vi "PvgeneratorOP300.vi"(8 "errin":errorcluster, 10 "network":path, 11 "path in":path) -> (0 "sortie d'erreur":errorcluster caption="errout", 1 "network out":path, 2 "tout bon":bool, 3 "Chaîne":string)   [LabVIEW 2020]
uses:
  VG/IS30%.vi
  VG/PN.vi
  <vilib>/Utility/config.llb/NI_LVConfig.lvlib
panel:
  out "nombre de remplacements":i32
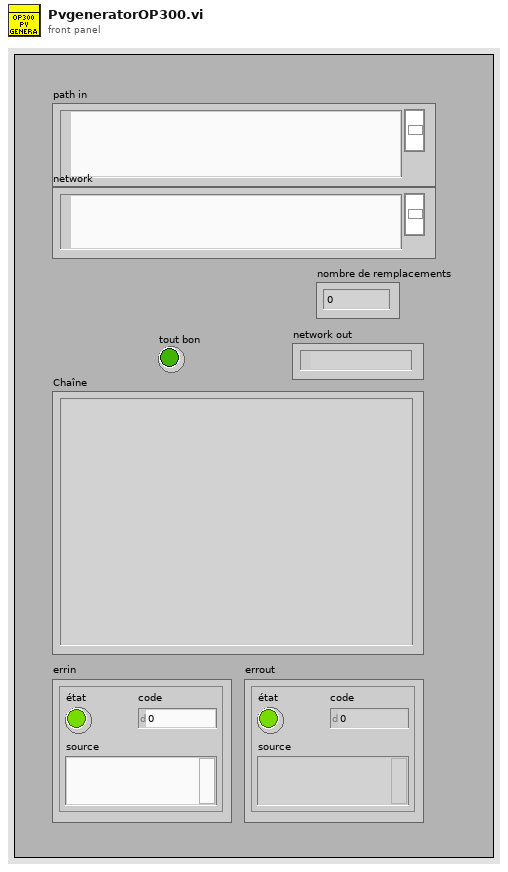
[diagram p1: front panel]
types:
  T1 = enum16{"open", "replace", "create", "open or create", "replace or create", "replace or create with confirmation"}
  T2 = typedef "NI_LVConfig.lvlib/Config Data RefNum.ctl" = refnum<k1>
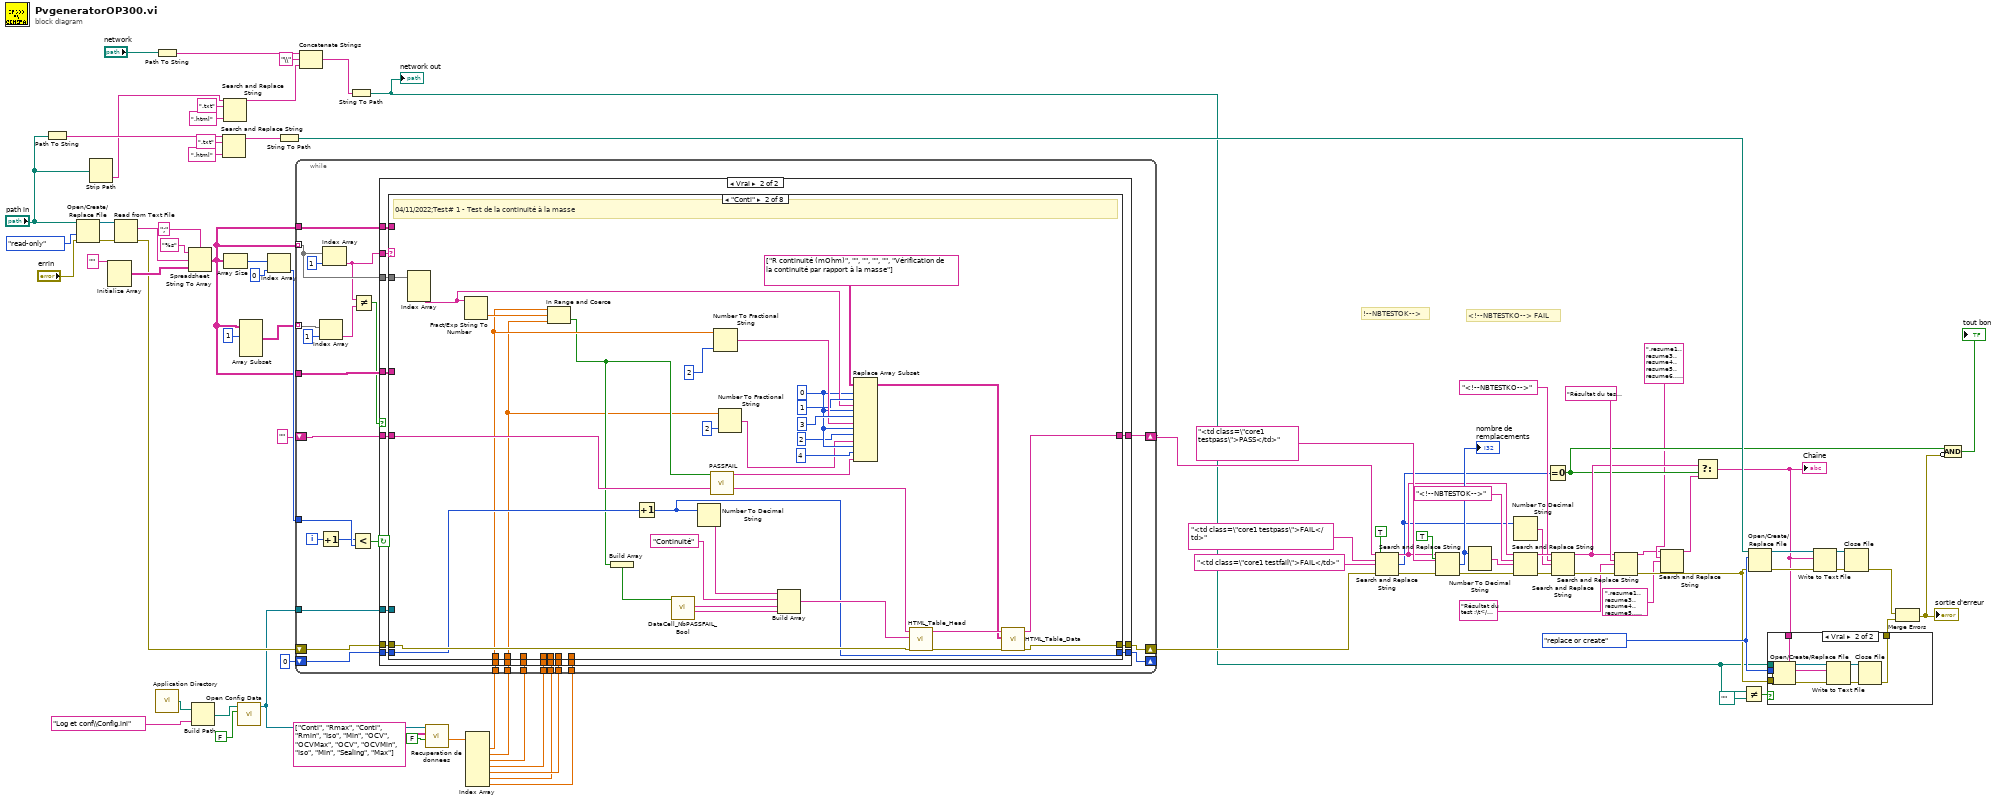
[diagram p0: block diagram]
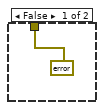
[diagram p2: hidden frame]
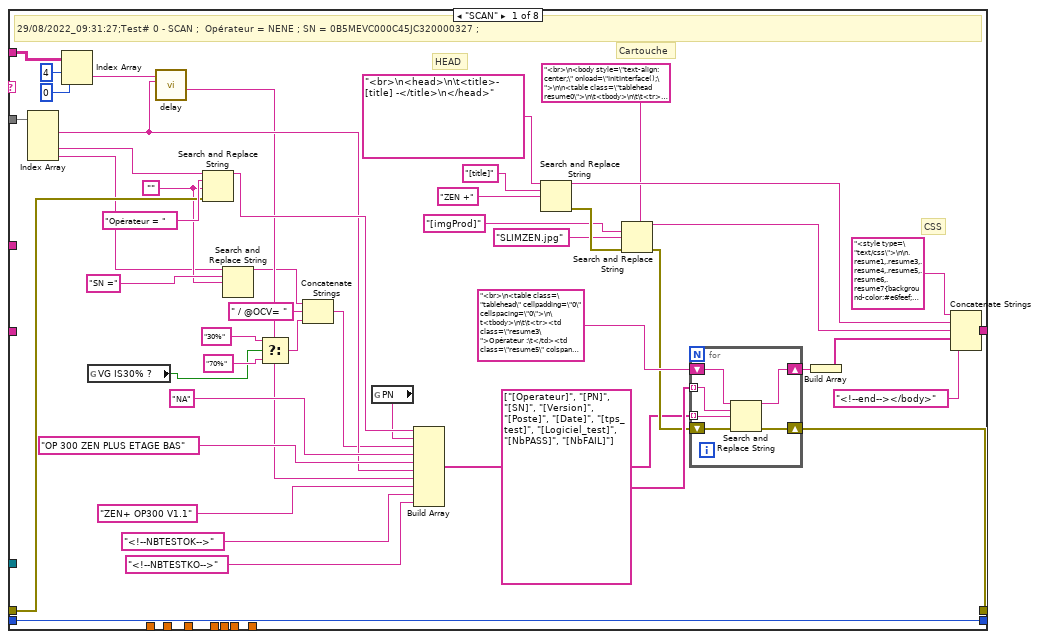
[diagram p4: hidden frame]
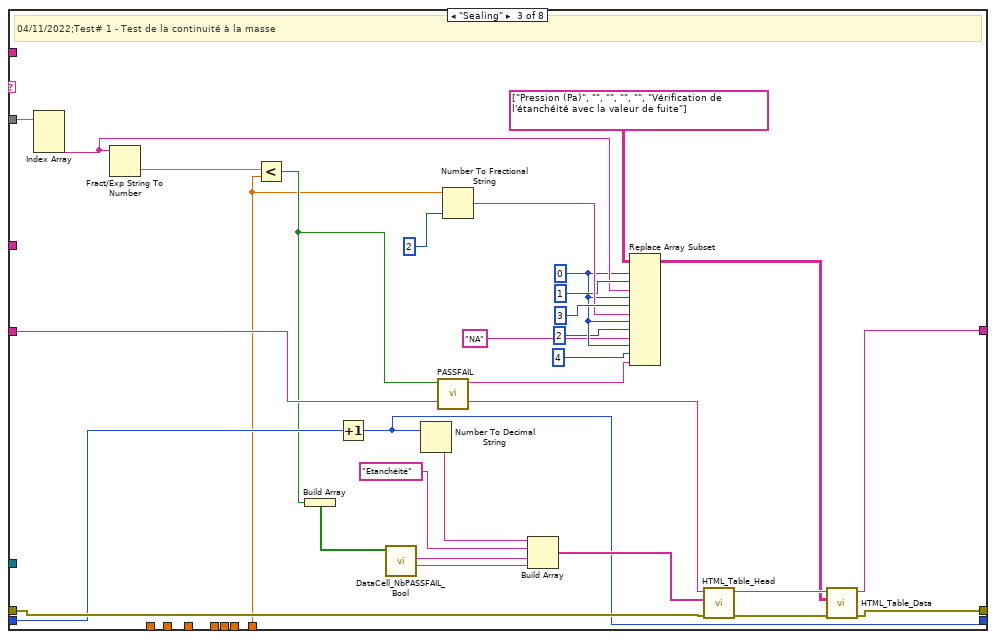
[diagram p5: hidden frame]
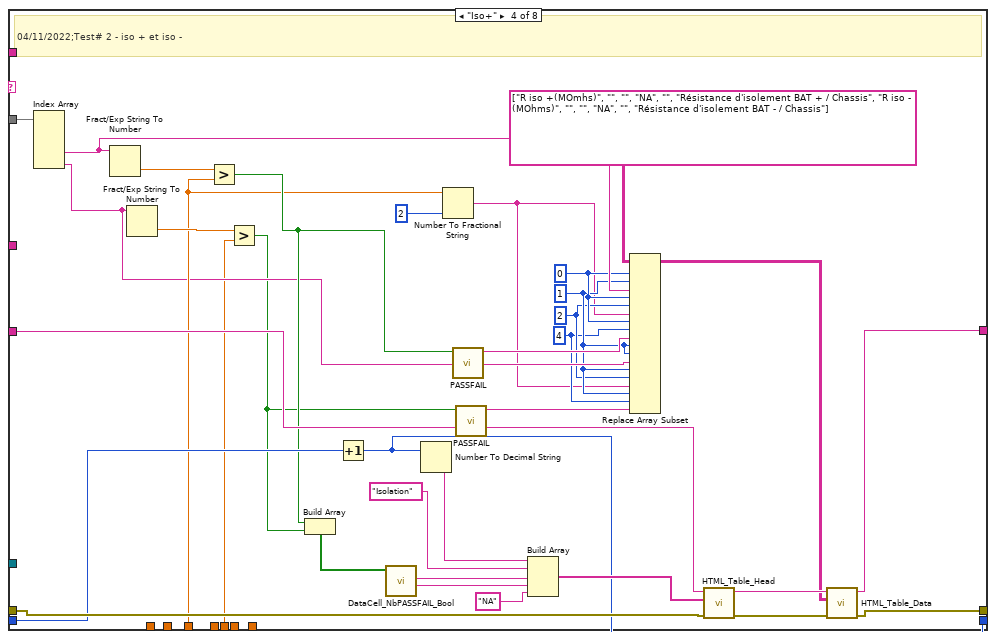
[diagram p6: hidden frame]
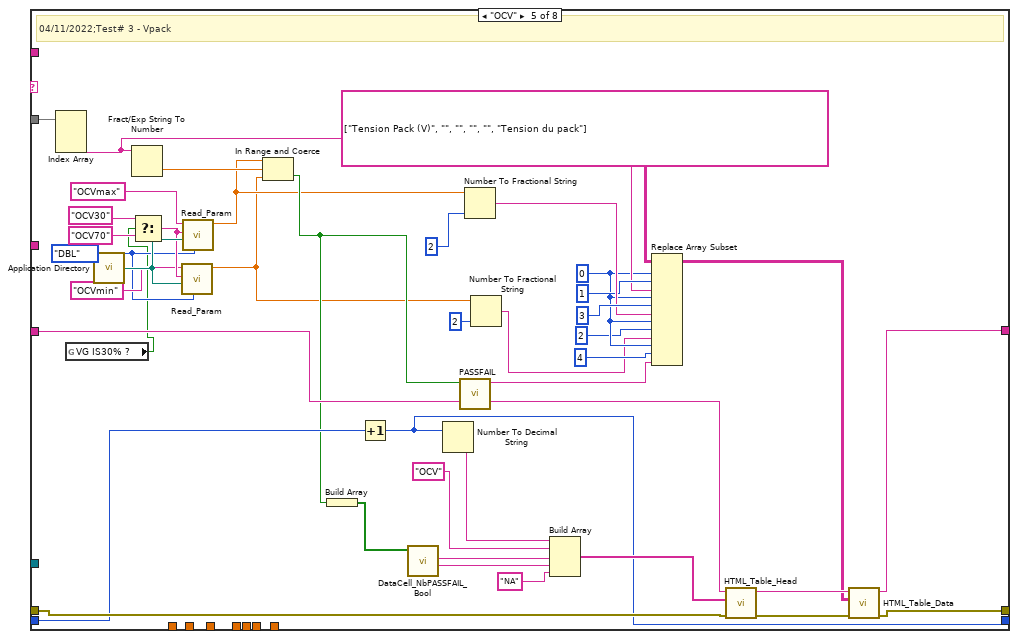
[diagram p7: hidden frame]
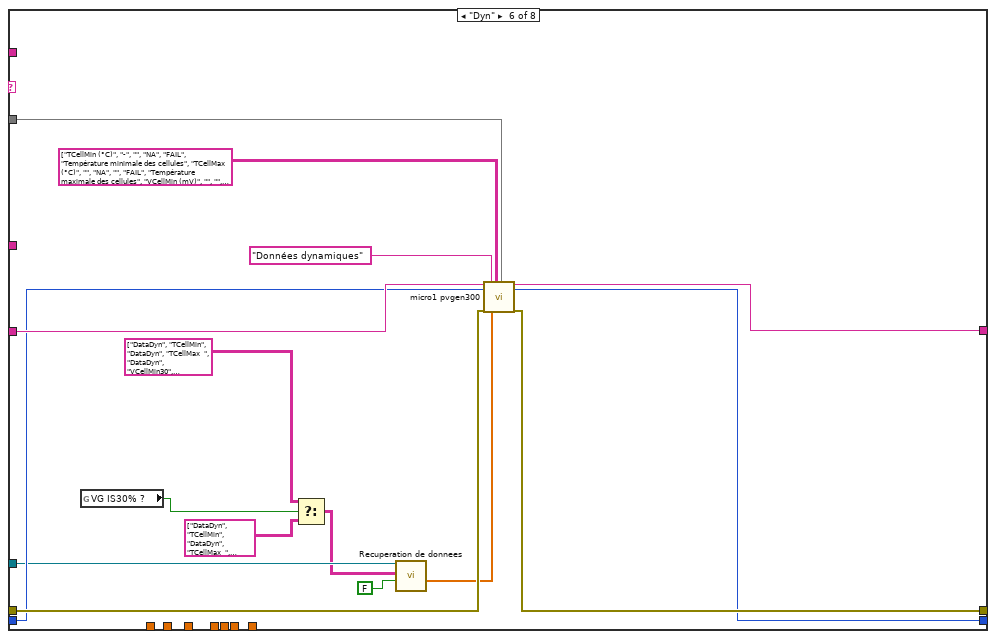
[diagram p8: hidden frame]
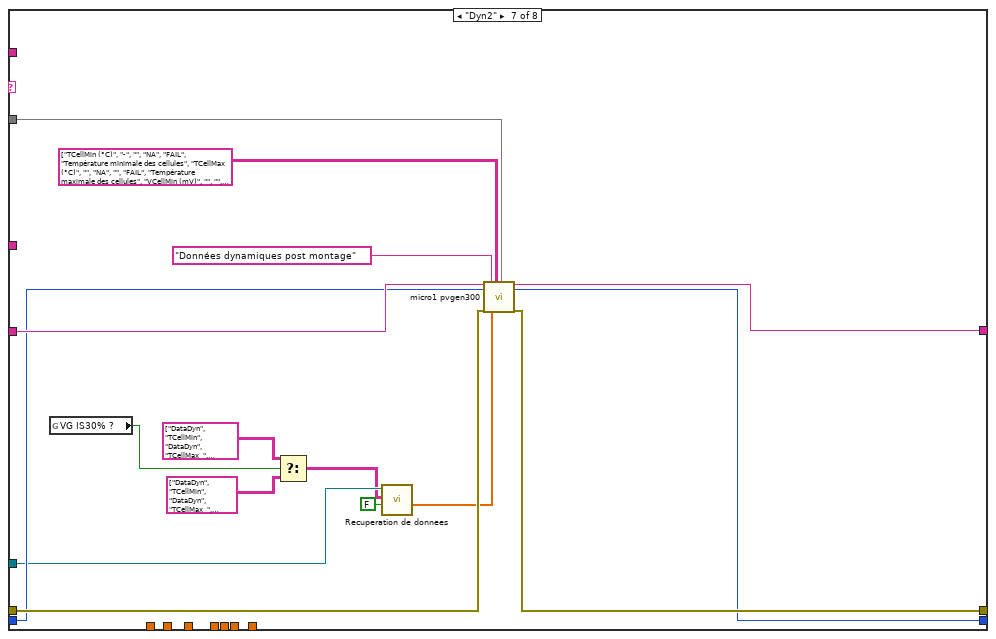
[diagram p9: hidden frame]
diagram:
  w47 = T1."replace or create" ("opération (0 : open)")
  # "<!--NBTESTKO--> FAIL"
  # "!--NBTESTOK-->"
  n1 = Path To String(path="path in") -> (string=w69:string)
  n2 = Open/Create/Replace File(file path (use dialog)="path in", error in="errin", access (0:read/write)=enum16{"read/write", "read-only", "write-only"}."read-only" ("accès (0 : read/write)")) -> (refnum out=w70:refnum<file>, error out=w87:errorcluster)  [unwired: 3 in, 1 out]
  n3 = Strip Path(path="path in") -> (name=w28:string)  [unwired: 1 out]
  n4 = Initialize Array("") -> (w85:string[][])  [unwired: 2 in]
  n5 = Read from Text File(file (use dialog)=w70, error in=w87) -> (text=w83:string, error out=w75:errorcluster)  [unwired: 2 in, 2 out]
  n6 = Path To String(path="network") -> (string=w27:string)
  n7 = call <vilib>:"Application Directory.vi"() -> ("Application Directory"=w19:path)
  n8 = Spreadsheet String To Array(delimiter (Tab)=";" ("séparateur (Tabulation)"), format string="%s" ("chaîne de format"), spreadsheet string=w83, array type (2D Dbl)=w85) -> (array=w6:string[][])
  n9 = Build Path(base path=w19, name or relative path="Log et conf\\Config.ini") -> (appended path=w22:path)
  n10 = Search and Replace String(input string=w69, search string=".txt" ("chaîne recherchée"), replace string=".html" ("chaîne de remplacement (\"\")")) -> (result string=w66:string)  [unwired: 5 in, 3 out]
  n11 = Search and Replace String(input string=w28, search string=".txt" ("chaîne recherchée"), replace string=".html" ("chaîne de remplacement (\"\")")) -> (result string=w25:string)  [unwired: 5 in, 3 out]
  n12 = Array Size(array=w6) -> (size(s)=w81:i32[])
  n13 = call <vilib>:"Open Config Data.vi"("create file if necessary (T)"=FALSE, "configuration file path"=w22) -> ("refnum"=w1:T2)  [unwired: 7 in, 2 out]
  n14 = Array Subset(array=w6, index (row)=1 ("indice")) -> (w4:string[][])  [unwired: 3 in]
  n15 = Index Array(array=w81, index=0 ("indice")) -> (element=w79:i32)
  n16 = String To Path(string=w66) -> (path=w65:path)
  n17 = Concatenate Strings(w27, "\\" ("chaîne"), w25) -> (w24:string)
  n18 = String To Path(string=w24) -> (path=w30:path)
  "network out" <- w30
  n19 = call "Recuperation de donnees.vi"("Est-ce un string?"=FALSE, "Array in"=string[][] [["Conti", "Rmax"], ["Conti", "Rmin"], ["Iso", "Min"], ["OCV", "OCVMax"], ["OCV", "OCVMin"], ["Iso", "Min"], ["Sealing", "Max"]], "Refnum in"=w1) -> ("Array"=w16:dbl[])  [unwired: 7 in, 1 out]
  n20 = Index Array(array=w16) -> (element #1=w15:dbl, element #2=w14:dbl, element #3=w13:dbl, element #4=w12:dbl, element #5=w11:dbl, element #6=w3:dbl, element #7=w2:dbl)  [unwired: 7 in]
  n21 = while {
    tunnel: w79 -> [w114]
    tunnel: w6 -> [w111] mode=indexing
    shift-right: [w110] -> w62
    shift-left: w75 -> [w109]
    shift-right: [w103] -> w64
    shift-left: "" -> [w108]
    shift-right: [w106] -> _
    shift-left: 0 -> [w107]
    tunnel: w6 -> [w105]
    tunnel: w15 -> [w102]
    tunnel: w14 -> [w101]
    tunnel: w6 -> [w100]
    tunnel: w13 -> [w99]
    tunnel: w12 -> [w98]
    tunnel: w11 -> [w97]
    tunnel: w4 -> [w95] mode=indexing
    tunnel: w3 -> [w91]
    tunnel: w2 -> [w90]
    tunnel: w1 -> [w89]
    i -> [w115]
    stop <- w113 continue-if-true
    n22 = Index Array(array=w95, index=1 ("indice")) -> (element=w94:string)
    n23 = Increment(x=w115) -> (x+1=w104:i32)
    n24 = Index Array(array=w111, index=1 ("indice")) -> (element=w93:string)
    n25 = Less?(x=w104, y=w114) -> (x < y?=w113:bool)
    n26 = Not Equal?(x=w93, y=w94) -> (x != y?=w92:bool)
    n27 = case shown="Vrai" w92 {
      tunnel: w111 -> [_ w136]
      tunnel: [w117 w135] -> w110
      tunnel: w109 -> [w117 w134]
      tunnel: w108 -> [w118 w133]
      tunnel: w107 -> [w116 w132]
      tunnel: [w116 w131] -> w106
      tunnel: w105 -> [_ w130]
      tunnel: [w118 w129] -> w103
      tunnel: w93 -> [_ w128]
      tunnel: w102 -> [_ w127]
      tunnel: w101 -> [_ w126]
      tunnel: w100 -> [_ w125]
      tunnel: w99 -> [_ w124]
      tunnel: w98 -> [_ w123]
      tunnel: w97 -> [_ w122]
      tunnel: w91 -> [_ w121]
      tunnel: w90 -> [_ w120]
      tunnel: w89 -> [_ w119]
      frame False {
      }
      frame True {
        n28 = case shown="\"Conti\"" w128 {
          tunnel: w134 -> [w181 w214 w244 w277 w318 w342 w358 w361]
          tunnel: w136 -> [w183 w215 w245 w278 w319 w339 w355 _]
          tunnel: [w160 w213 w243 w276 w317 w341 w357 w361] -> w135
          tunnel: w133 -> [_ w212 w242 w275 w316 w338 w354 w359]
          tunnel: w132 -> [w159 w211 w241 w274 w315 w337 w353 w360]
          tunnel: [w159 w210 w240 w273 w314 w336 w352 w360] -> w131
          tunnel: w130 -> [_ _ _ _ _ _ _ _]
          tunnel: [w158 w209 w239 w272 w313 w340 w356 w359] -> w129
          tunnel: w127 -> [_ w198 _ _ _ _ _ _]
          tunnel: w126 -> [_ w191 _ _ _ _ _ _]
          tunnel: w125 -> [w151 _ _ _ _ _ _ _]
          tunnel: w124 -> [_ _ _ w261 _ _ _ _]
          tunnel: w123 -> [_ _ _ _ _ _ _ _]
          tunnel: w122 -> [_ _ _ _ _ _ _ _]
          tunnel: w121 -> [_ _ _ w252 _ _ _ _]
          tunnel: w120 -> [_ _ w222 _ _ _ _ _]
          tunnel: w119 -> [_ _ _ _ _ w335 w351 _]
          frame "SCAN" {
            w154 = ""
            # "Cartouche"
            # "HEAD"
            # "CSS"
            # "29/08/2022_09:31:27;Test# 0 - SCAN ;  Opérateur = NENE ; SN = 0B5MEVC000C45JC320000327 ;"
            n29 = Index Array(array=w183) -> (element #1=w147:string, element #3=w157:string, element #4=w152:string)  [unwired: 4 in, 1 out]
            n30 = Index Array(array=w151, index (row)=4, index (col)=0 ("disabled index (col)")) -> (element=w148:string)
            n31 = global read "IS30%.vi" "VG IS30% ?"() -> (w138:bool)
            n32 = call "delay.vi"("String"=w147, "String 2"=w148) -> ("Delay calculé"=w146:string)  [unwired: 9 in]
            n33 = Search and Replace String(input string=w157, search string="Opérateur = " ("chaîne recherchée"), replace string=w154, error in=w181) -> (result string=w156:string)  [unwired: 4 in, 3 out]
            n34 = Search and Replace String(input string=w152, search string="SN =" ("chaîne recherchée"), replace string=w154) -> (result string=w144:string)  [unwired: 5 in, 3 out]
            n35 = Select(t="30%" ("y"), s=w138, f="70%" ("y")) -> (s? t:f=w141:string)
            n36 = Concatenate Strings(w144, " / @OCV= " ("chaîne"), w141) -> (w143:string)
            n37 = global read "PN.vi" "PN"() -> (w137:string)
            n38 = Build Array(w156, w137, w143, "NA" ("element"), "OP 300 ZEN PLUS ETAGE BAS" ("chaîne"), w147, w146, "ZEN+ OP300 V1.1" ("chaîne"), "<!--NBTESTOK-->" ("chaîne"), "<!--NBTESTKO-->" ("chaîne")) -> (w161:string[])
            n39 = Search and Replace String(input string="<br>\n<head>\n\t<title>- [title] -</title>\n</head>", search string="[title]" ("chaîne recherchée"), replace string="ZEN +" ("Title")) -> (result string=w177:string, error out=w176:errorcluster)  [unwired: 5 in, 2 out]
            n40 = Search and Replace String(input string="<br>\n<body style=\"text-align: center;\" onload=\"InitInterface();\">\n\n<table class=\"tablehead resume0\">\n\t<tbody>\n\t\t<tr>\n\t\t\t<td> <img src=\"[imgProd]\" style=\"width:194px;height:100px\" class=\"left\"></td>\n\t\t\t<td> <div class=\"center\">PROCES VERBAL DE TEST AUTOMATIQUE</div><div class=\"center\">Zen Plus OP 300</div><br class=\"center\"><div class=\"center\">Forseepower</div></td>\n\t\t\t<td> <img src=\"LOGO FORSEE.png\" style=\"width:194px;height:100px\"  class=\"right\"></td>\n\t\t</tr>\n\t</tbody>\n</table>", search string="[imgProd]", replace string="SLIMZEN.jpg" ("imgProd"), error in=w176) -> (result string=w174:string, error out=w171:errorcluster)  [unwired: 4 in, 2 out]
            n41 = for {
              shift-right: [w188] -> w170
              shift-left: "<br>\n<table class=\"tablehead\" cellpadding=\"0\" cellspacing=\"0\">\n\t<tbody>\n\t\t<tr><td class=\"resume3\">Opérateur :\t</td><td class=\"resume5\" colspan=\"3\">[Operateur]</td></tr>\n\t\t<tr><td class=\"resume3\">PN : </td><td class=\"resume5\" colspan=\"3\">[PN]</td></tr>\n\t\t<tr><td class=\"resume3\">SN : </td><td class=\"resume5\" colspan=\"3\">[SN]</td></tr>\n\t\t<tr><td class=\"resume3\">Version : </td><td class=\"resume5\" colspan=\"3\">[Version]</td></tr>\n\t\t<tr><td class=\"resume3\">Poste : </td><td class=\"resume5\" colspan=\"3\">[Poste]</td></tr>\t\t\n\t\t<tr><td class=\"resume3\">Date du test : </td><td class=\"resume5\" colspan=\"3\">[Date]</td></tr>\n\t\t<tr><td class=\"resume3\">Temps de test : </td><td class=\"resume5\" colspan=\"3\">[tps_test]</td></tr>\n\t\t<tr><td class=\"resume3\">Logiciel de test :\t</td><td class=\"resume5\" colspan=\"3\">[Logiciel_test]</td></tr>\n\t\t<tr><td class=\"resume3\">Résultat du test :\t</td><td class=\"resume5\" colspan=\"3\"><div><span style=\"float:left\" id=\"result\"><font size = \"5pt\" color=\"green\"><b>CONFORME</b></font><b><font size = \"5pt\"> ( </font><font size = \"5pt\" color=\"green\">[NbPASS] PASS </font>  <font size = \"5pt\"> / </font><font size = \"5pt\" color=\"red\">[NbFAIL] FAIL</font> <font size = \"5pt\"> ) </font></b></span></div></td></tr>\n\t</tbody>\n</table>" -> [w189]
              tunnel: string[] ["[Operateur]", "[PN]", "[SN]", "[Version]", "[Poste]", "[Date]", "[tps_test]", "[Logiciel_test]", "[NbPASS]", "[NbFAIL]"] -> [w185] mode=indexing
              tunnel: w161 -> [w184] mode=indexing
              shift-right: [w186] -> w160
              shift-left: w171 -> [w187]
              n42 = Search and Replace String(input string=w189, search string=w185, replace string=w184, error in=w187) -> (result string=w188:string, error out=w186:errorcluster)  [unwired: 4 in, 2 out]
            }
            n43 = Build Array(w170) -> (w169:string[])
            n44 = Concatenate Strings("<style type=\"text/css\">\n\n.resume1,.resume3,.resume4,.resume5,.resume6,.resume7{background-color:#e6feef;padding:7px;border:1px solid black;}\n.resume0{border:1px solid black;background-color:#e6feef;font-weight: bold;padding:0px;text-align: center;}\n.resume1{width:350px;text-align:right;font-weight:bold;}\n.resume3{width:350px;text-align:right;border-top:0px solid black;font-weight:bold;}\n.resume4{border-left:0px solid black;width:290px;}\n.resume5{width:290px;border-left:0px solid black;border-top:0px solid black;}\n.resume6{border-left:0px solid black;width:60px;}\n.resume7{border-left:0px solid black;border-top:0px solid black;width:60px;}\n.title1{text-align: left;background-color:#e6f4fe;padding:10px;border:1px solid #101010;}\n.title2{width: 30px;text-align: center;background-color:#e6f4fe;padding:1px;border:1px solid #101010;border-left:0px solid black;font-weight: bold;}\n.title2 a:link{text-decoration:none;}\n.entete0,.entete1,.entete2,.time2{text-align: center;background-color:#feeec9;padding:7px;border:1px solid black;font-weight: bold;}\n.entete0{width:45px;border-right:0px solid black;}\n.entete1{width:505px;}\n.entete2{width:95px;border-right:0px solid black;}\n.time2{border-left:0px solid black;width:145px;font-size:11px;}\n.core0,.core1,.core2,.core3,.core4,.time{text-align: center;background-color:#fafed3;padding:7px;border:1px solid black;}\n.core0, .core1,.core3,.core4{width:95px;border-top:0px solid black;border-right:0px solid black;}\n.core0{width:45px;}\n.core2{border-top:0px solid black;width:505px;}\n.core3{width:200px;}\n.core4{width:300px;}\n.time{width:145px;border-top:0px solid black;border-left:0px solid black;font-size:11px;}\n.false .core0,.false .core1,.false .core2,.false .core3,.false .core4,.false .time{background-color:#f4f4f4;}\n.false .entete0,.false .entete1,.false .entete2,.false .time2{background-color:#dadada;}\n.false .title1,.false .title2,.false .resultentete .testpass,.false .resultentete .testfail,.false .resultentete .testtime{background-color:#c5cac9;color: blue;}\n.false .title2 a:link{text-decoration:none;color: blue;}\n.comment1,.comment2,.time3{width: 890px;background-color:#e9e8e9;padding:7px;border:1px solid black;border-top:0px solid black;text-align:left;}\n.comment2{border-right:0px solid black;width: 45px;text-align: center;}\n.time3{width: 145px;border-left:0px solid black;font-size:11px;}\n.fixe1{background: -moz-linear-gradient(center top , #101010 10%, #555555 80%) repeat scroll 0 0 transparent;background: -webkit-gradient(linear, left top, left bottom, from(#101010), to(#555555));border:2px solid orange;position : fixed;margin-top:20px;display:none;overflow-y:scroll;max-height:350px;text-shadow: 0px 0px 0 #333333;text-align:left;font-size:10px;padding:10px;margin-left:-162px;border-radius: 15px 15px 15px 15px;}\n.menufixe, .menufixelock{background: -moz-linear-gradient(center top , #101010 80%, transparent 20%) repeat scroll 0 0 transparent;background: -webkit-gradient(linear, left top, left bottom, from(#101010), color-stop(0.65, #101010), to(transparent)) repeat scroll 0 0 transparent;margin: -52px 0px 0px -9px;width:100%;position:fixed;height:55px;-moz-transition: margin 1s;-webkit-transition: margin 1s;}\n.menufixelock, .menufixe:hover{margin: -9px 0px 0px -9px;}\n.lockmenu, .separation,.separationmenu{text-align:center;background: -moz-linear-gradient(center top , #555555 10%, #111111 80%) repeat scroll 0 0 transparent;background: -webkit-gradient(linear, left top, left bottom, from(#555555), to(#111111));border: 1px solid white;border-radius: 10px 10px 10px 10px;box-shadow: 0 -1px 1px #555555 inset;color: #999999;font-weight: bold;width: 100px;padding: 2px;text-decoration: none;}\n.tablehead{width: 1000px;font-family: Verdana;font-size: 12px;margin-left: auto;margin-right: auto;}\n.tablenull{font-family: Verdana;font-size: 11px;margin-left: auto;margin-right: auto;}\n.separationmenu:hover div{display: inline;}\n.lockmenu:hover, .separation:hover,.separationmenu:hover{border: 1px solid orange;cursor:pointer;}\n.lockmenu:hover{border: 1px solid red;cursor:pointer;}\n.separationright{padding:10px;}\ndiv a:link{text-decoration:none;color:#cbcbcb;}\ndiv a:hover{text-decoration:underline;color:#cbcbcb;}\nspan a:link{text-decoration:none;color:#cbcbcb;}\nspan a:hover{text-decoration:none;color:#cbcbcb;}\n.false{color: blue;}\n.testpass{color: green;font-weight: bold;}\n.testfail{color: red;font-weight: bold;}\n.testtime{color: blue;font-weight: bold;}\n.resultentete{font-weight: bold;font-size: 11px;min-width: 200px;text-align:right;}\n.infohard{border: 1px solid black;background-color: white;text-align: center;width: 16px;height: 16px;border-radius: 5px;font-weight: bold;box-shadow: 0 -1px 2px #555555 inset;}\n.infohard:hover{background-color:#feeec9;cursor:pointer;}\n.footerhard{padding-top:30px;}\n.confighard{font-size:10px;width:110px;}\n.circlemain{margin-left:auto;margin-right:auto;}\n.circletext,.circleform{padding-top: 3px;text-align:center;font-size: 10px;width:200px;}\n.circleform{padding-bottom: 3px;padding-top: 1px;}\n.circle{border: 1px solid black;border-collapse: collapse;border-radius: 15px;box-shadow: 1px 1px 0 #505050;height: 15px;width: 15px;display:inline-block;}\n.bookmarkon, .bookmarkoff{background-color: yellow;border: 1px solid black;border-collapse: collapse;border-radius: 10px 10px 10px 10px;box-shadow: 1px 1px 0 #505050;height: 12px;width: 12px;position: absolute;margin-left:22px;cursor: help;}\n.bookmarkoff{background-color: transparent;border: 1px solid #CECECE;box-shadow: none;cursor: copy;}\n.false .bookmarkoff{background-color: transparent;border: 1px solid #E6E1E1;box-shadow: none;cursor: copy;}\n.bookmarkmaster{height: 15px;margin-right: 12px;width: 60px;}\n.bookmarkmaster:hover .bookmarkprev,.bookmarkmaster:hover .bookmarksuiv{display:block;}\n.bookmarkprev, .bookmarksuiv {cursor: pointer;font-size: 25px;font-weight: bold;margin-top: -10px;position: absolute;display:none;}\n.bookmarkprev{margin-left: 2px;}\n.bookmarksuiv{margin-left: 43px;}\n.plus, .moins{background-color: #F4F4F4;border: 1px solid #848484;border-radius: 20px;color: #848484;font-family: arial;font-size: 16px;font-weight: bold;height: 20px;margin-left: 4px;text-align: center;width: 20px;}\n.moins{font-size: 15px;}\n.plus:hover, .moins:hover{background-color: #DADADA;border: 1px solid black;color: black;cursor:pointer;}\n.backtothetop {position: fixed; right: 50%; margin-right: -555px; bottom: 10px; font-size: 35px; font-weight: bold; border: 1px solid #7D7B91; width: 40px; height: 40px; line-height:52px; text-align: center;border-radius: 8px; opacity: 0.25; background-color: #F5F5F5; color:#7D7B91;}\n.backtothetop:hover {opacity: 1; cursor:pointer;}\n.libversion {font-size: 8px;font-weight: normal;padding-right: 10px;text-align: right;}\n.lockmenu {width: 18px;font-size: 12px;}\n.left {display: block; margin-left: 1px;margin-right: auto;}\n.right {display: block; margin-right: 1px;margin-left: auto;}\n.center {display: block; margin-left: auto;margin-right: auto;}\n\n</style>", w177, w174, w169, "<!--end--></body>") -> (w158:string)
          }
          frame "Conti" {
            w195 = 0 ("index (row)")
            # "04/11/2022;Test# 1 - Test de la continuité à la masse"
            n45 = Index Array(array=w215) -> (element #3=w200:string)  [unwired: 3 in, 2 out]
            n46 = Fract/Exp String To Number(string=w200) -> (number=w199:dbl)  [unwired: 3 in, 1 out]
            n47 = In Range and Coerce(upper limit=w198, x=w199, lower limit=w191) -> (In Range?=w193:bool)  [unwired: 1 out]
            n48 = Build Array(w193) -> (w207:bool[])
            n49 = Increment(x=w211) -> (x+1=w210:i32)
            n50 = call <vilib>:"DataCell_NbPASSFAIL_Bool.vi"("Tableau en entrée"=w207) -> ("Chaîne"=w205:string, "Chaîne 2"=w206:string)  [unwired: 8 in, 1 out]
            n51 = Number To Decimal String(number=w210) -> (decimal integer string=w217:string)  [unwired: 1 in]
            n52 = call <vilib>:"PASSFAIL.vi"("E"=w193) -> ("S"=w197:string)  [unwired: 10 in]
            n53 = Number To Fractional String(number=w198, precision (6)=i16 2) -> (F-format string=w203:string)  [unwired: 2 in]
            n54 = Number To Fractional String(number=w191, precision (6)=i16 2) -> (F-format string=w190:string)  [unwired: 2 in]
            n55 = Build Array(w217, "Continuité" ("élément"), w206, w205) -> (w220:string[])
            n56 = Replace Array Subset(array=string[][] [["R continuité (mOhm)", "", "", "", "", "Vérification de la continuité par rapport à la masse"]] ("Tableau"), new element #1=w200, index (row) #1=w195, index (col) #1=1 ("disabled index (col)"), new element #2=w203, index (row) #2=w195, index (col) #2=3 ("disabled index (col)"), new element #3=w190, index (row) #3=w195, index (col) #3=2 ("disabled index (col)"), new element #4=w197, index (row) #4=w195, index (col) #4=4 ("disabled index (col)")) -> (w208:string[][])
            n57 = call "HTML_Table_Head.vi"("entrée d'erreur (pas d'erreur)"=w214, "Tableau"=w220, "chaîne en entrée"=w212) -> ("sortie d'erreur"=w219:errorcluster, "result string"=w218:string)  [unwired: 7 in]
            n58 = call "HTML_Table_Data.vi"("entrée d'erreur (pas d'erreur)"=w219, "Tableau"=w208, "chaîne en entrée"=w218) -> ("sortie d'erreur"=w213:errorcluster, "result string"=w209:string)  [unwired: 7 in]
          }
          frame "Sealing" {
            w226 = 0 ("index (row)")
            # "04/11/2022;Test# 1 - Test de la continuité à la masse"
            n59 = Index Array(array=w245) -> (element #3=w230:string)  [unwired: 3 in, 2 out]
            n60 = Fract/Exp String To Number(string=w230) -> (number=w229:dbl)  [unwired: 3 in, 1 out]
            n61 = Less?(x=w229, y=w222) -> (x < y?=w224:bool)
            n62 = Build Array(w224) -> (w237:bool[])
            n63 = Increment(x=w241) -> (x+1=w240:i32)
            n64 = call <vilib>:"DataCell_NbPASSFAIL_Bool.vi"("Tableau en entrée"=w237) -> ("Chaîne"=w235:string, "Chaîne 2"=w236:string)  [unwired: 8 in, 1 out]
            n65 = Number To Decimal String(number=w240) -> (decimal integer string=w247:string)  [unwired: 1 in]
            n66 = call <vilib>:"PASSFAIL.vi"("E"=w224) -> ("S"=w228:string)  [unwired: 10 in]
            n67 = Number To Fractional String(number=w222, precision (6)=i16 2) -> (F-format string=w233:string)  [unwired: 2 in]
            n68 = Build Array(w247, "Etanchéité" ("élément"), w236, w235) -> (w250:string[])
            n69 = Replace Array Subset(array=string[][] [["Pression (Pa)", "", "", "", "", "Vérification de l'étanchéité avec la valeur de fuite"]] ("Tableau"), new element #1=w230, index (row) #1=w226, index (col) #1=1 ("disabled index (col)"), new element #2=w233, index (row) #2=w226, index (col) #2=3 ("disabled index (col)"), new element #3="NA" ("nouvel élément/sous-tableau"), index (row) #3=w226, index (col) #3=2 ("disabled index (col)"), new element #4=w228, index (row) #4=w226, index (col) #4=4 ("disabled index (col)")) -> (w238:string[][])
            n70 = call "HTML_Table_Head.vi"("entrée d'erreur (pas d'erreur)"=w244, "Tableau"=w250, "chaîne en entrée"=w242) -> ("sortie d'erreur"=w249:errorcluster, "result string"=w248:string)  [unwired: 7 in]
            n71 = call "HTML_Table_Data.vi"("entrée d'erreur (pas d'erreur)"=w249, "Tableau"=w238, "chaîne en entrée"=w248) -> ("sortie d'erreur"=w243:errorcluster, "result string"=w239:string)  [unwired: 7 in]
          }
          frame "Iso+" {
            w256 = 4 ("disabled index (col)")
            w257 = 2 ("disabled index (col)")
            w258 = 1 ("disabled index (col)")
            w265 = 0 ("index (row)")
            # "04/11/2022;Test# 2 - iso + et iso -"
            n72 = Index Array(array=w278) -> (element #3=w266:string, element #5=w259:string)  [unwired: 5 in, 3 out]
            n73 = Fract/Exp String To Number(string=w266) -> (number=w264:dbl)  [unwired: 3 in, 1 out]
            n74 = Fract/Exp String To Number(string=w259) -> (number=w262:dbl)  [unwired: 3 in, 1 out]
            n75 = Greater?(x=w264, y=w261) -> (0:w263:bool)
            n76 = Greater?(x=w262, y=w252) -> (0:w254:bool)
            n77 = Build Array(w263, w254) -> (w270:bool[])
            n78 = Increment(x=w274) -> (x+1=w273:i32)
            n79 = call <vilib>:"DataCell_NbPASSFAIL_Bool.vi"("Tableau en entrée"=w270) -> ("Chaîne"=w268:string, "Chaîne 2"=w269:string)  [unwired: 8 in, 1 out]
            n80 = Number To Decimal String(number=w273) -> (decimal integer string=w281:string)  [unwired: 1 in]
            n81 = Number To Fractional String(number=w261, precision (6)=i16 2) -> (F-format string=w255:string)  [unwired: 2 in]
            n82 = call <vilib>:"PASSFAIL.vi"("E"=w263) -> ("S"=w260:string)  [unwired: 10 in]
            n83 = call <vilib>:"PASSFAIL.vi"("E"=w254) -> ("S"=w253:string)  [unwired: 10 in]
            n84 = Build Array(w281, "Isolation" ("élément"), w269, w268, "NA" ("élément")) -> (w284:string[])
            n85 = Replace Array Subset(array=string[][] [["R iso +(MOmhs)", "", "", "NA", "", "Résistance d'isolement BAT + / Chassis"], ["R iso - (MOhms)", "", "", "NA", "", "Résistance d'isolement BAT - / Chassis"]] ("Tableau"), new element #1=w266, index (row) #1=w265, index (col) #1=w258, new element #2=w255, index (row) #2=w265, index (col) #2=w257, new element #3=w260, index (row) #3=w265, index (col) #3=w256, new element #4=w259, index (row) #4=w258, index (col) #4=w258, new element #5=w255, index (row) #5=w258, index (col) #5=w257, new element #6=w253, index (row) #6=w258, index (col) #6=w256) -> (w271:string[][])
            n86 = call "HTML_Table_Head.vi"("entrée d'erreur (pas d'erreur)"=w277, "Tableau"=w284, "chaîne en entrée"=w275) -> ("sortie d'erreur"=w283:errorcluster, "result string"=w282:string)  [unwired: 7 in]
            n87 = call "HTML_Table_Data.vi"("entrée d'erreur (pas d'erreur)"=w283, "Tableau"=w271, "chaîne en entrée"=w282) -> ("sortie d'erreur"=w276:errorcluster, "result string"=w272:string)  [unwired: 7 in]
          }
          frame "OCV" {
            w289 = enum16{"STR", "DBL", "U32"}."DBL" ("Énum")
            w300 = 0 ("index (row)")
            # "04/11/2022;Test# 3 - Vpack"
            n88 = Index Array(array=w319) -> (element #3=w304:string)  [unwired: 3 in, 2 out]
            n89 = global read "IS30%.vi" "VG IS30% ?"() -> (w286:bool)
            n90 = call <vilib>:"Application Directory.vi"() -> ("Application Directory"=w293:path)
            n91 = Fract/Exp String To Number(string=w304) -> (number=w303:dbl)  [unwired: 3 in, 1 out]
            n92 = Select(t="OCV30" ("section"), s=w286, f="OCV70" ("section")) -> (s? t:f=w292:string)
            n93 = call "Read_Param.vi"("Énum"=w289, "pathin"=w293, "section"=w292, "key"="OCVmin") -> ("dbl"=w287:dbl)  [unwired: 3 in, 4 out]
            n94 = call "Read_Param.vi"("Énum"=w289, "pathin"=w293, "section"=w292, "key"="OCVmax") -> ("dbl"=w288:dbl)  [unwired: 3 in, 4 out]
            n95 = In Range and Coerce(upper limit=w288, x=w303, lower limit=w287) -> (In Range?=w298:bool)  [unwired: 1 out]
            n96 = Build Array(w298) -> (w311:bool[])
            n97 = Increment(x=w315) -> (x+1=w314:i32)
            n98 = call <vilib>:"DataCell_NbPASSFAIL_Bool.vi"("Tableau en entrée"=w311) -> ("Chaîne"=w309:string, "Chaîne 2"=w310:string)  [unwired: 8 in, 1 out]
            n99 = Number To Decimal String(number=w314) -> (decimal integer string=w322:string)  [unwired: 1 in]
            n100 = call <vilib>:"PASSFAIL.vi"("E"=w298) -> ("S"=w302:string)  [unwired: 10 in]
            n101 = Number To Fractional String(number=w288, precision (6)=i16 2) -> (F-format string=w307:string)  [unwired: 2 in]
            n102 = Number To Fractional String(number=w287, precision (6)=i16 2) -> (F-format string=w296:string)  [unwired: 2 in]
            n103 = Build Array(w322, "OCV" ("élément"), w310, w309, "NA" ("élément")) -> (w325:string[])
            n104 = Replace Array Subset(array=string[][] [["Tension Pack (V)", "", "", "", "", "Tension du pack"]] ("Tableau"), new element #1=w304, index (row) #1=w300, index (col) #1=1 ("disabled index (col)"), new element #2=w307, index (row) #2=w300, index (col) #2=3 ("disabled index (col)"), new element #3=w296, index (row) #3=w300, index (col) #3=2 ("disabled index (col)"), new element #4=w302, index (row) #4=w300, index (col) #4=4 ("disabled index (col)")) -> (w312:string[][])
            n105 = call "HTML_Table_Head.vi"("entrée d'erreur (pas d'erreur)"=w318, "Tableau"=w325, "chaîne en entrée"=w316) -> ("sortie d'erreur"=w324:errorcluster, "result string"=w323:string)  [unwired: 7 in]
            n106 = call "HTML_Table_Data.vi"("entrée d'erreur (pas d'erreur)"=w324, "Tableau"=w312, "chaîne en entrée"=w323) -> ("sortie d'erreur"=w317:errorcluster, "result string"=w313:string)  [unwired: 7 in]
          }
          frame "Dyn" {
            n107 = global read "IS30%.vi" "VG IS30% ?"() -> (w328:bool)
            n108 = Select(t=string[][] [["DataDyn", "TCellMin"], ["DataDyn", "TCellMax  "], ["DataDyn", "VCellMin30"], ["DataDyn", "VCellMax30"], ["DataDyn", "TusineMax"], ["DataDyn", "TusineMin"], ["DataDyn", "DeltaT "], ["DataDyn", "DeltaV "]], s=w328, f=string[][] [["DataDyn", "TCellMin"], ["DataDyn", "TCellMax  "], ["DataDyn", "VCellMin70 "], ["DataDyn", "VCellMax70"], ["DataDyn", "TusineMax"], ["DataDyn", "TusineMin"], ["DataDyn", "DeltaT "], ["DataDyn", "DeltaV "]]) -> (s? t:f=w329:string[][])
            n109 = call "Recuperation de donnees.vi"("Est-ce un string?"=FALSE, "Array in"=w329, "Refnum in"=w335) -> ("Array"=w331:dbl[])  [unwired: 7 in, 1 out]
            n110 = call "micro1 pvgen300.vi"("FluxStrIn"=w338, "Numin"=w337, "errin"=w342, "testlabel"="Données dynamiques", "Data limit"=w331, "tab ref"=string[][] [["TCellMin (°C)", "-", "", "NA", "FAIL", "Température minimale des cellules"], ["TCellMax (°C)", "", "NA", "", "FAIL", "Température maximale des cellules"], ["VCellMin (mV)", "", "", "NA", "FAIL", "Tension minimale des cellues"], ["VCellMax (mV)", "", "NA", "", "FAIL", "Tension maximale des cellues"], ["Tusine (°C)", "", "", "", "FAIL", "Température de l'usine"], ["DeltaT (°C)", "", "NA", "", "FAIL", "Différence maximale de température entre les cellules"], ["DeltaV  (mV)", "", "NA", "", "FAIL", "Différence maximale de tension entre les cellules"]] ("Tableau"), "ligne à traiter"=w339) -> ("result string"=w340:string, "Numout"=w336:i32, "errout"=w341:errorcluster)  [unwired: 10 in]
          }
          frame "Dyn2" {
            n111 = global read "IS30%.vi" "VG IS30% ?"() -> (w343:bool)
            n112 = Select(t=string[][] [["DataDyn", "TCellMin"], ["DataDyn", "TCellMax  "], ["DataDyn", "VCellMin30"], ["DataDyn", "VCellMax30"], ["DataDyn", "TusineMax"], ["DataDyn", "TusineMin"], ["DataDyn", "DeltaT "], ["DataDyn", "DeltaV "]], s=w343, f=string[][] [["DataDyn", "TCellMin"], ["DataDyn", "TCellMax  "], ["DataDyn", "VCellMin70 "], ["DataDyn", "VCellMax70"], ["DataDyn", "TusineMax"], ["DataDyn", "TusineMin"], ["DataDyn", "DeltaT "], ["DataDyn", "DeltaV "]]) -> (s? t:f=w345:string[][])
            n113 = call "Recuperation de donnees.vi"("Est-ce un string?"=FALSE, "Array in"=w345, "Refnum in"=w351) -> ("Array"=w344:dbl[])  [unwired: 7 in, 1 out]
            n114 = call "micro1 pvgen300.vi"("FluxStrIn"=w354, "Numin"=w353, "errin"=w358, "testlabel"="Données dynamiques post montage", "Data limit"=w344, "tab ref"=string[][] [["TCellMin (°C)", "-", "", "NA", "FAIL", "Température minimale des cellules"], ["TCellMax (°C)", "", "NA", "", "FAIL", "Température maximale des cellules"], ["VCellMin (mV)", "", "", "NA", "FAIL", "Tension minimale des cellues"], ["VCellMax (mV)", "", "NA", "", "FAIL", "Tension maximale des cellues"], ["Tusine (°C)", "", "", "", "FAIL", "Température de l'usine"], ["DeltaT (°C)", "", "NA", "", "FAIL", "Différence maximale de température entre les cellules"], ["DeltaV  (mV)", "", "NA", "", "FAIL", "Différence maximale de tension entre les cellules"]] ("Tableau"), "ligne à traiter"=w355) -> ("result string"=w356:string, "Numout"=w352:i32, "errout"=w357:errorcluster)  [unwired: 10 in]
          }
          frame "NULL", Default {
            # "NULL"
          }
        }
      }
    }
  }
  n115 = Search and Replace String(replace all?=TRUE ("tout remplacer ? (F)"), input string=w64, search string="<td class=\"core1 testpass\">FAIL</td>" ("chaîne recherchée"), replace string="<td class=\"core1 testfail\">FAIL</td>" ("chaîne de remplacement (\"\")"), error in=w62) -> (result string=w48:string, number of replacements=w43:i32, error out=w59:errorcluster)  [unwired: 3 in, 1 out]
  n116 = Search and Replace String(replace all?=TRUE ("tout remplacer ? (F)"), input string=w48, search string="<td class=\"core1 testpass\">PASS</td>" ("chaîne recherchée"), error in=w59) -> (number of replacements=w51:i32, error out=w55:errorcluster)  [unwired: 4 in, 2 out]
  "nombre de remplacements" <- w51
  n117 = Number To Decimal String(number=w51) -> (decimal integer string=w50:string)  [unwired: 1 in]
  n118 = Number To Decimal String(number=w43) -> (decimal integer string=w49:string)  [unwired: 1 in]
  n119 = Search and Replace String(input string=w48, search string="<!--NBTESTOK-->" ("chaîne recherchée"), replace string=w50, error in=w55) -> (result string=w56:string, error out=w54:errorcluster)  [unwired: 4 in, 2 out]
  n120 = Equal To 0?(x=w43) -> (x = 0?=w35:bool)
  n121 = Search and Replace String(input string=w56, search string="<!--NBTESTKO-->" ("chaîne recherchée"), replace string=w49, error in=w54) -> (result string=w38:string, error out=w42:errorcluster)  [unwired: 4 in, 2 out]
  n122 = Search and Replace String(input string=w38, search string="Résultat du test :\t</td><td class=\"resume5\" colspan=\"3\"><div><span style=\"float:left\" id=\"result\"><font size = \"5pt\" color=\"green\"><b>CONFORME</b>", replace string="Résultat du test :\t</td><td class=\"resume5\" colspan=\"3\"><div><span style=\"float:left\" id=\"result\"><font  size = \"5pt\" color=\"red\"><b>NON CONFORME</b>", error in=w42) -> (result string=w8:string, error out=w41:errorcluster)  [unwired: 4 in, 2 out]
  n123 = Search and Replace String(input string=w8, search string=".resume1,.resume3,.resume4,.resume5,.resume6,.resume7{background-color:#e6feef;padding:7px;border:1px solid black;}\n.resume0{border:1px solid black;background-color:#e6feef;font-weight: bold;padding:0px;text-align: center;}", replace string=".resume1,.resume3,.resume4,.resume5,.resume6,.resume7{background-color:#fdebd0;padding:7px;border:1px solid black;}\n.resume0{border:1px solid black;background-color:#fdebd0;font-weight: bold;padding:0px;text-align: center;}") -> (result string=w7:string)  [unwired: 5 in, 3 out]
  n124 = Select(t=w38, s=w35, f=w7) -> (s? t:f=w39:string)
  "Chaîne" <- w39
  n125 = Not Equal?(x=w30, y=path "") -> (x != y?=w32:bool)
  n126 = Open/Create/Replace File(file path (use dialog)=w65, error in=w41, operation (0:open)=w47) -> (refnum out=w71:refnum<file>, error out=w73:errorcluster)  [unwired: 3 in, 1 out]
  n127 = case shown="Vrai" w32 {
    tunnel: w47 -> [_ w367]
    tunnel: w30 -> [_ w366]
    tunnel: w41 -> [_ w365]
    tunnel: w39 -> [_ w364]
    tunnel: [errorcluster {"status"=FALSE, "code"=0, "source"=""} ("error out") w363] -> w37
    frame False {
    }
    frame True {
      n128 = Open/Create/Replace File(file path (use dialog)=w366, error in=w365, operation (0:open)=w367) -> (refnum out=w368:refnum<file>, error out=w370:errorcluster)  [unwired: 3 in, 1 out]
      n129 = Write to Text File(file (use dialog)=w368, text=w364, error in=w370) -> (refnum out=w369:refnum<file>, error out=w371:errorcluster)  [unwired: 1 in, 1 out]
      n130 = Close File(refnum=w369, error in=w371) -> (error out=w363:errorcluster)  [unwired: 1 out]
    }
  }
  n131 = Write to Text File(file (use dialog)=w71, text=w39, error in=w73) -> (refnum out=w72:refnum<file>, error out=w74:errorcluster)  [unwired: 1 in, 1 out]
  n132 = Close File(refnum=w72, error in=w74) -> (error out=w36:errorcluster)  [unwired: 1 out]
  n133 = Merge Errors(w36, w37) -> (w34:errorcluster)
  "sortie d'erreur" <- w34
  n134 = Compound Arithmetic op=AND ("Opérateur arithmétique")(w35, invert w34) -> (→"tout bon":bool)
